vi "启动流程.vi"   [LabVIEW 2022 SP3, in "重金属.lvlib"]
types:
  T1 = cluster{"时间标识":timestamp, "设备":string, "日志信息":string, "流程参数":string}
  T2 = cluster{"时间标识":timestamp, "测量模式":string, "数据类型":string, "监测值":sgl, "单位":string, "数据标识":string, "因子编码":string, "标样参考值":sgl}
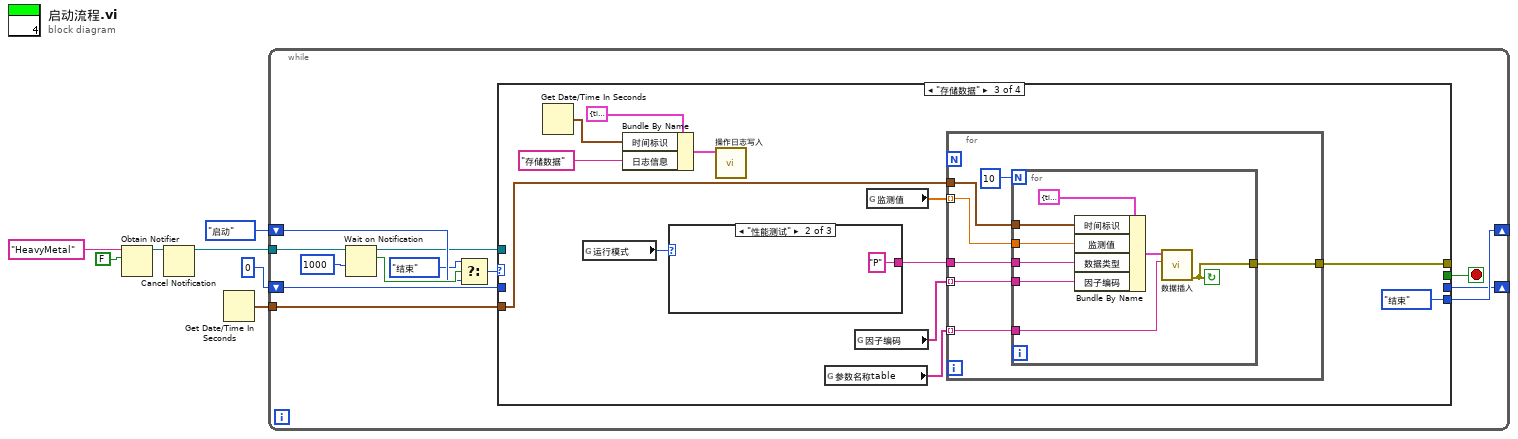
[diagram p0: block diagram]
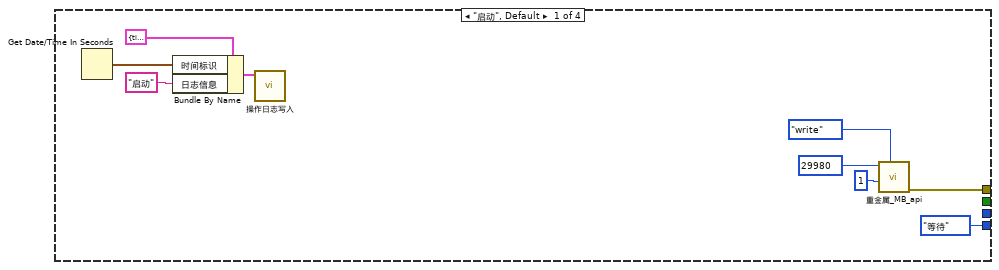
[diagram p2: hidden frame]
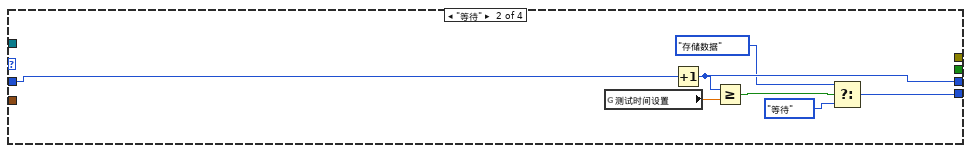
[diagram p3: hidden frame]
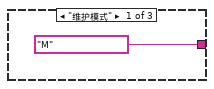
[diagram p4: hidden frame]
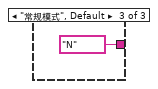
[diagram p5: hidden frame]
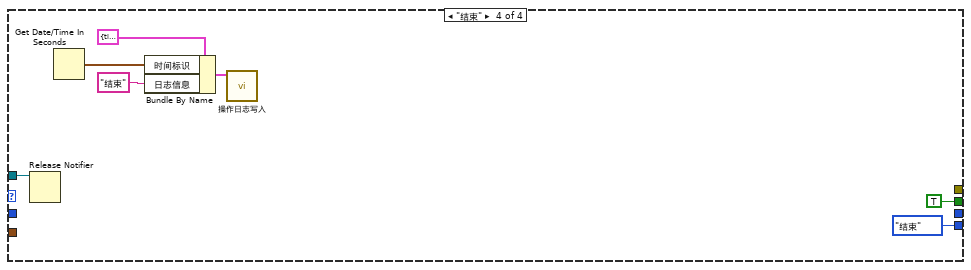
[diagram p6: hidden frame]
diagram:
  n1 = Obtain Notifier(name (unnamed)="HeavyMetal" ("名称（未命名）"), notification data type=FALSE) -> (notifier out=w2:refnum<notifier>)  [unwired: 2 in, 2 out]
  n2 = Cancel Notification(0:w2) -> (8:w1:refnum<notifier>)  [unwired: 1 in, 2 out]
  n3 = Get Date/Time In Seconds() -> (seconds since 1Jan1904=w5:timestamp)
  n4 = while {
    shift-right: [w19] -> _
    shift-left: enum16{"启动", "等待", "存储数据", "结束"}."启动" ("枚举") -> [w11]
    shift-right: [w17] -> _
    shift-left: u32 0 ("等待时间（毫秒）") -> [w18]
    tunnel: w5 -> [w15]
    tunnel: w1 -> [w14]
    stop <- w16 stop-if-true
    n5 = Wait on Notification(notifier=w14, timeout in ms (-1)=1000 ("超时毫秒(-1)")) -> (notifier out=w8:refnum<notifier>, notification=w12:bool)  [unwired: 2 in, 2 out]
    n6 = Select(t=enum16{"启动", "等待", "存储数据", "结束"}."结束", s=w12, f=w11) -> (s? t:f=w10:enum16{"启动", "等待", "存储数据", "结束"})
    n7 = case shown="\"存储数据\"" w10 {
      tunnel: [w25 _ w40 _] -> _
      tunnel: [enum16{"启动", "等待", "存储数据", "结束"}."等待" ("枚举") w31 enum16{"启动", "等待", "存储数据", "结束"}."结束" ("枚举") enum16{"启动", "等待", "存储数据", "结束"}."结束" ("枚举")] -> w19
      tunnel: w18 -> [_ w35 _ _]
      tunnel: [_ w34 _ _] -> w17
      tunnel: [_ _ _ TRUE] -> w16
      tunnel: w15 -> [_ _ w39 _]
      tunnel: w8 -> [_ _ _ w66]
      frame "启动", Default {
        n8 = Get Date/Time In Seconds() -> (seconds since 1Jan1904=w21:timestamp)
        n9 = Bundle By Name(cluster=T1 {"时间标识"=timestamp(0 s since 1904-01-01), "设备"="重金属", "日志信息"="", "流程参数"=""} ("data in"), "时间标识"=w21, "日志信息"="启动") -> (w22:T1)
        n10 = call "操作日志写入.vi"("data in"=w22) -> ()  [unwired: 10 in, 1 out]
        n11 = call "重金属_MB_api.vi"("STEP"=enum16{"open", "read", "write", "close"}."write", "values"=u16 1, "starting address"=u16 29980) -> ("error out"=w25:errorcluster)  [unwired: 5 in, 3 out]
      }
      frame "等待" {
        n12 = global read "全局变量.vi" "测试时间设置"() -> (w29:dbl)
        n13 = Increment(x=w35) -> (x+1=w34:u32)
        n14 = Greater Or Equal?(x=w34, y=w29) -> (x >= y?=w33:bool)
        n15 = Select(t=enum16{"启动", "等待", "存储数据", "结束"}."存储数据" ("枚举"), s=w33, f=enum16{"启动", "等待", "存储数据", "结束"}."等待" ("枚举")) -> (s? t:f=w31:enum16{"启动", "等待", "存储数据", "结束"})
      }
      frame "存储数据" {
        n16 = Get Date/Time In Seconds() -> (seconds since 1Jan1904=w44:timestamp)
        n17 = global read "全局变量.vi" "运行模式"() -> (w41:enum16{"维护模式", "常规模式", "应急模式", "质控模式", "性能测试"})
        n18 = Bundle By Name(cluster=T1 {"时间标识"=timestamp(0 s since 1904-01-01), "设备"="重金属", "日志信息"="", "流程参数"=""} ("data in"), "时间标识"=w44, "日志信息"="存储数据") -> (w45:T1)
        n19 = case shown="\"性能测试\"" w41 {
          tunnel: ["M" ("数据标记表") "P" ("数据标记表") "N" ("数据标记表")] -> w42
          frame "维护模式" {
          }
          frame "性能测试" {
          }
          frame "常规模式", Default {
          }
        }
        n20 = call "操作日志写入.vi"("data in"=w45) -> ()  [unwired: 10 in, 1 out]
        n21 = global read "全局变量.vi" "参数名称table"() -> (w38:string[])
        n22 = global read "全局变量.vi" "因子编码"() -> (w37:string[])
        n23 = global read "全局变量.vi" "监测值"() -> (w36:dbl[])
        n24 = for {
          tunnel: w36 -> [w56] mode=indexing
          tunnel: w42 -> [w57]
          tunnel: [w55] -> w40
          tunnel: w39 -> [w54]
          tunnel: w37 -> [w53] mode=indexing
          tunnel: w38 -> [w52] mode=indexing
          n25 = for {
            N: 10 -> [_]
            tunnel: w57 -> [w65]
            tunnel: w56 -> [w64]
            tunnel: [w58] -> w55
            tunnel: w54 -> [w63]
            tunnel: w53 -> [w62]
            tunnel: w52 -> [w61]
            stop <- w58 continue-if-true
            n26 = Bundle By Name(cluster=T2 {"时间标识"=timestamp(0 s since 1904-01-01), "测量模式"="水样测试", "数据类型"="N", "监测值"=0.0, "单位"="mg/L", "数据标识"="N", "因子编码"="w20122", "标样参考值"=0.0} ("data"), "时间标识"=w63, "监测值"=w64, "数据类型"=w65, "因子编码"=w62) -> (w60:T2)
            n27 = call "数据插入.vi"("table"=w61, "data"=w60) -> ("error out"=w58:errorcluster)  [unwired: 9 in]
          }
        }
      }
      frame "结束" {
        n28 = Release Notifier(notifier=w66) -> ()  [unwired: 2 in, 3 out]
        n29 = Get Date/Time In Seconds() -> (seconds since 1Jan1904=w68:timestamp)
        n30 = Bundle By Name(cluster=T1 {"时间标识"=timestamp(0 s since 1904-01-01), "设备"="重金属", "日志信息"="", "流程参数"=""} ("data in"), "时间标识"=w68, "日志信息"="结束") -> (w69:T1)
        n31 = call "操作日志写入.vi"("data in"=w69) -> ()  [unwired: 10 in, 1 out]
      }
    }
  }
